vi "读取数据文件-拉伸.vi"(0 "文件路径（使用对话框）":path) -> (1 "第一列":dbl[](array[numeric]), 2 "第二列":dbl[](array[numeric]))   [LabVIEW 2016]
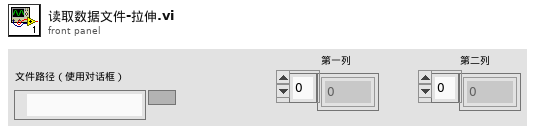
[diagram p1: front panel]
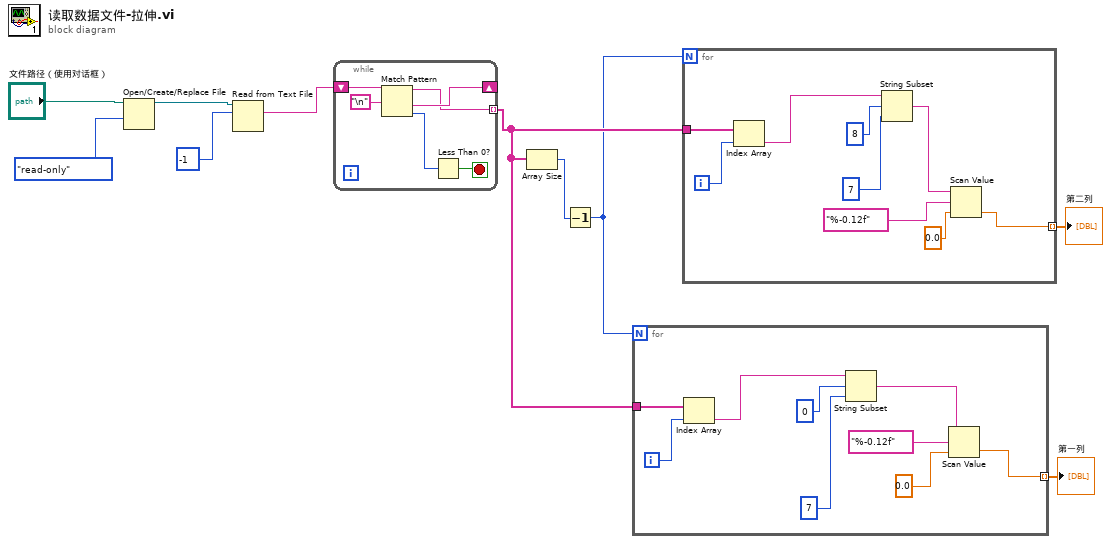
[diagram p0: block diagram]
diagram:
  n1 = Open/Create/Replace File(file path (use dialog)="文件路径（使用对话框）", access (0:read/write)=enum16{"read/write", "read-only", "write-only"}."read-only" ("权限(0:read/write)")) -> (refnum out=w8:refnum<file>)  [unwired: 4 in, 2 out]
  n2 = Read from Text File(file (use dialog)=w8, count=-1 ("计数")) -> (text=w6:string)  [unwired: 2 in, 3 out]
  n3 = while {
    tunnel: [w11] -> w4 mode=indexing
    shift-right: [w14] -> _
    shift-left: w6 -> [w15]
    stop <- w13 stop-if-true
    n4 = Match Pattern(string=w15, regular expression="\n") -> (before substring=w11:string, after substring=w14:string, offset past match=w12:i32)  [unwired: 1 in, 1 out]
    n5 = Less Than 0?(x=w12) -> (x < 0?=w13:bool)
  }
  n6 = Array Size(array=w4) -> (size(s)=w5:i32)
  n7 = Decrement(x=w5) -> (x-1=w3:i32)
  n8 = for {
    N: w3 -> [_]
    tunnel: w4 -> [w25]
    tunnel: [w17] -> w1 mode=indexing
    i -> [w24]
    n9 = Index Array(array=w25, index=w24) -> (element=w23:string)
    n10 = String Subset(string=w23, offset (0)=0 ("偏移量(0)"), length (rest)=7 ("长度（剩余）")) -> (substring=w18:string)
    n11 = Scan Value(string=w18, format string="%-0.12f" ("格式字符串"), default (0 dbl)=0.0 ("默认(0 dbl)")) -> (value=w17:dbl)  [unwired: 1 out]
  }
  "第一列" <- w1
  n12 = for {
    N: w3 -> [_]
    tunnel: w4 -> [w34]
    tunnel: [w26] -> w2 mode=indexing
    i -> [w33]
    n13 = Index Array(array=w34, index=w33) -> (element=w32:string)
    n14 = String Subset(string=w32, offset (0)=8 ("偏移量(0)"), length (rest)=7 ("长度（剩余）")) -> (substring=w29:string)
    n15 = Scan Value(string=w29, format string="%-0.12f" ("格式字符串"), default (0 dbl)=0.0 ("默认(0 dbl)")) -> (value=w26:dbl)  [unwired: 1 out]
  }
  "第二列" <- w2
